vi "Find FlatSequence.vi"(8 "error in (no error)":errorcluster, 9 "i in":i32, 11 "VI in":refnum<vi>) -> (0 "error out":errorcluster, 1 "i out":i32, 3 "FlatSequences":T1[](array[typedef]))   [LabVIEW 2023, in "VIDoc Parsing.lvlib" / "Structure Reporter.lvlib"]
uses:
  Structure Reporter.lvlib
  Structure Result 2.ctl
  <vilib>/Utility/traverseref.llb/TRef TravTarget.ctl
  <vilib>/Utility/traverseref.llb/VI Scripting - Traverse.lvlib
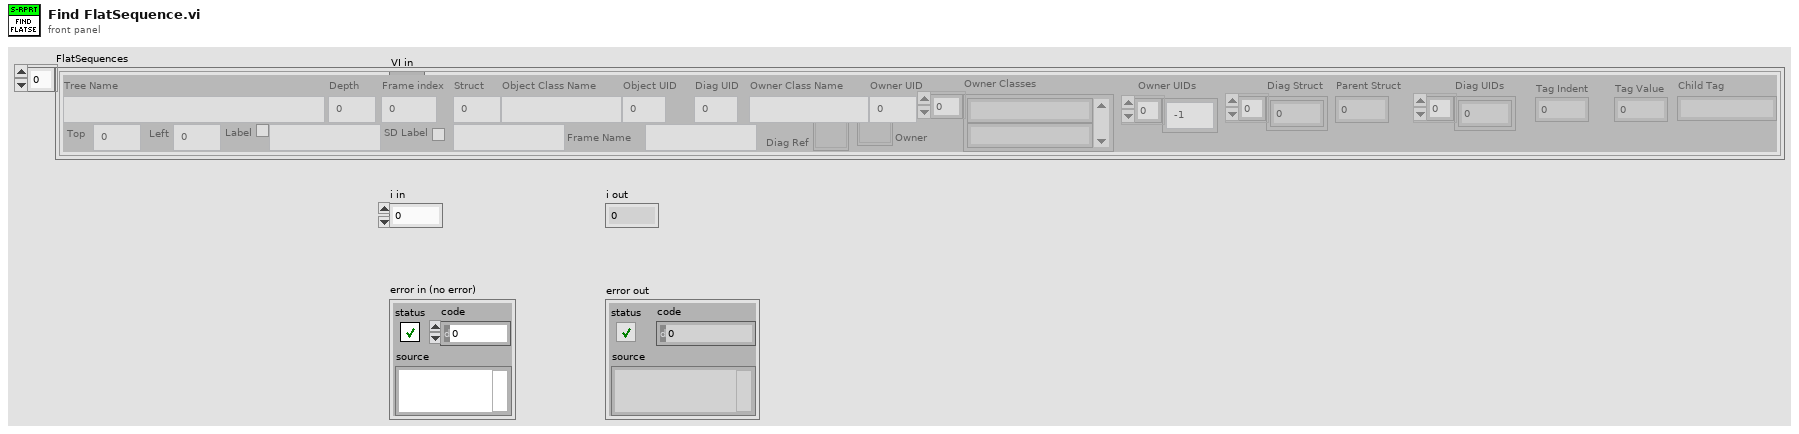
[diagram p1: front panel]
types:
  T1 = typedef "VIDoc Parsing.lvlib/Structure Reporter.lvlib/Structure Result 2.ctl" = cluster{"Depth":i32, "Top":i32, "Left":i32, "Frame index":i32, "Struct":i32, "Object Class Name":string, "Object UID":i32, "Label Visible":bool, "Object Label":string, "SD Label Visible":bool, "Object SD Label":string, "Frame Name":string, "Diag UID":i32, "Owner Class Name":string, "Owner UID":i32, "Diag Struct":i32[], "Parent Struct":i32, "Diag UIDs":i32[], "Tree Name":string, "Diag Ref":refnum<vi>, "Owner Classes":string[], "Owner":refnum<vi>, "Owner UIDs":i32[], "Tag Indent":i32, "Tag Value":i32, "Child Tag":string}
  T2 = typedef "TRef TravTarget.ctl" = enum16{"FP", "BD", "Other"}
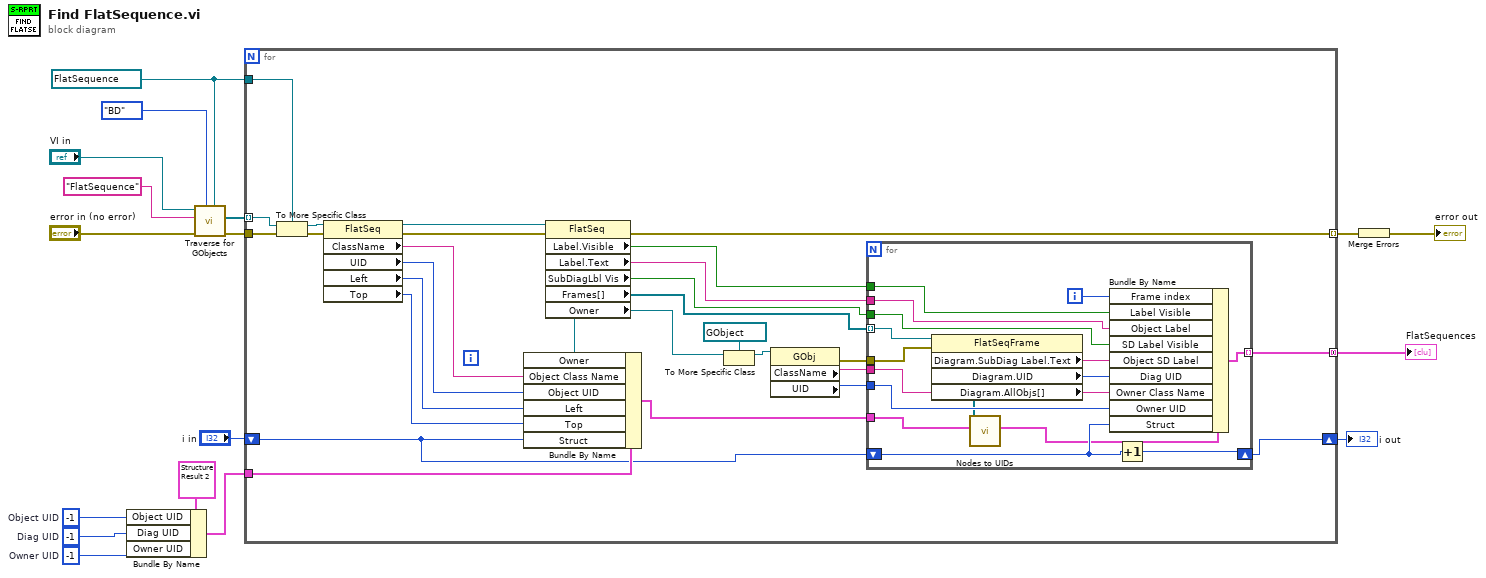
[diagram p0: block diagram]
diagram:
  w2 = -1  # Owner UID
  w3 = -1  # Diag UID
  w4 = -1  # Object UID
  w13 = refnum<vi> refnum ("Other Refnum")
  n1 = Bundle By Name(cluster=T1 {"Depth"=0, "Top"=0, "Left"=0, "Frame index"=0, "Struct"=0, "Object Class Name"="", "Object UID"=0, "Label Visible"=FALSE, "Object Label"="", "SD Label Visible"=FALSE, "Object SD Label"="", "Frame Name"="", "Diag UID"=0, "Owner Class Name"="", "Owner UID"=0, "Diag Struct"=[], "Parent Struct"=0, "Diag UIDs"=[], "Tree Name"="", "Diag Ref"=refnum, "Owner Classes"=[], "Owner"=refnum, "Owner UIDs"=[], "Tag Indent"=0, "Tag Value"=0, "Child Tag"=""}, "Object UID"=w4, "Diag UID"=w3, "Owner UID"=w2) -> (w1:T1)
  n2 = call <vilib>:"Traverse for GObjects.vi"("Other Refnum"=w13, "Traverse Target"=TRef_TravTarget."BD", "error in (no error)"="error in (no error)", "Class Name"="FlatSequence", "VI Refnum"="VI in") -> ("error out"=w16:errorcluster, "References"=w12:refnum<vi>[])  [unwired: 3 in, 2 out]
  n3 = for {
    tunnel: w12 -> [w42] mode=indexing
    tunnel: w13 -> [w41]
    tunnel: w1 -> [w40]
    tunnel: [w24] -> w14 mode=concatenating
    tunnel: w16 -> [w23]
    tunnel: [w21] -> w17 mode=indexing
    shift-right: [w19] -> w6
    shift-left: "i in" -> [w20]
    n4 = To More Specific Class(target class=w41, reference=w42, error in=w23) -> (specific class reference=w43:refnum<vi>, error out=w44:errorcluster)
    n5 = property class="FlatSeq"(reference=w43, error in=w44) -> (reference out=w26:refnum<vi>, error out=w22:errorcluster, "ClassName"=w39:string, "UID"=w38:i32, "Left"=w37:i32, "Top"=w36:i32)
    n6 = property class="FlatSeq"(reference=w26, error in=w22) -> (error out=w21:errorcluster, "Label.Visible"=w35:bool, "Label.Text"=w30:string, "SubDiagLbl Vis"=w29:bool, "Frames[]"=w27:refnum<vi>[], "Owner"=w18:refnum<vi>)  [unwired: 1 out]
    n7 = Bundle By Name(cluster=w40, "Owner"=w18, "Object Class Name"=w39, "Object UID"=w38, "Left"=w37, "Top"=w36, "Struct"=w20) -> (w25:T1)
    n8 = To More Specific Class(target class=refnum<vi> refnum ("Other Refnum"), reference=w18) -> (specific class reference=w33:refnum<vi>)  [unwired: 1 in, 1 out]
    n9 = property class="GObj"(reference=w33) -> (error out=w28:errorcluster, "ClassName"=w32:string, "UID"=w31:i32)  [unwired: 1 in, 1 out]
    n10 = for {
      tunnel: w35 -> [w60]
      tunnel: w32 -> [w55]
      tunnel: w31 -> [w54]
      tunnel: w30 -> [w59]
      tunnel: w29 -> [w58]
      tunnel: [w53] -> w24 mode=indexing
      tunnel: w28 -> [w52]
      tunnel: w27 -> [w51] mode=indexing
      tunnel: w25 -> [w46]
      shift-right: [w48] -> w19
      shift-left: w20 -> [w49]
      i -> [w50]
      n11 = property class="FlatSeqFrame"(reference=w51, error in=w52) -> ("Diagram.SubDiag Label.Text"=w57:string, "Diagram.UID"=w56:i32, "Diagram.AllObjs[]"=w47:refnum<vi>[])  [unwired: 2 out]
      n12 = call "Nodes to UIDs.vi"("cluster"=w46, "All Objects[]"=w47) -> ("Nodes"=w45:T1)  [unwired: 9 in]
      n13 = Bundle By Name(cluster=w45, "Frame index"=w50, "Label Visible"=w60, "Object Label"=w59, "SD Label Visible"=w58, "Object SD Label"=w57, "Diag UID"=w56, "Owner Class Name"=w55, "Owner UID"=w54, "Struct"=w49) -> (w53:T1)
      n14 = Increment(x=w49) -> (x+1=w48:i32)
    }
  }
  "FlatSequences" <- w14
  "i out" <- w6
  n15 = Merge Errors(w17) -> (→"error out":errorcluster)
